vi "Get First Elements From Arrays.vi"(9 "Pole-zero ratios":dbl[](array[numeric]), 10 "Compensation frequencies":dbl[](array[numeric]), 11 "Gain bandwidths":dbl[](array[numeric])) -> (1 "Pole-zero ratio":dbl, 2 "Compensation frequency":dbl, 3 "Gain bandwidth":dbl)   [LabVIEW 2021]
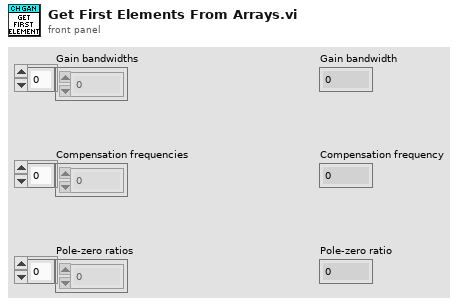
[diagram p1: front panel]
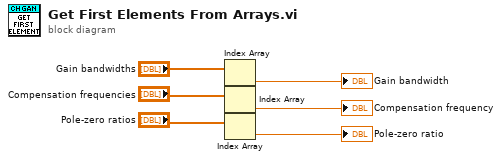
[diagram p0: block diagram]
diagram:
  n1 = Index Array(array="Gain bandwidths") -> (element=→"Gain bandwidth":dbl)  [unwired: 1 in]
  n2 = Index Array(array="Compensation frequencies") -> (element=→"Compensation frequency":dbl)  [unwired: 1 in]
  n3 = Index Array(array="Pole-zero ratios") -> (element=→"Pole-zero ratio":dbl)  [unwired: 1 in]
